vi "GUI Final add.vi"() -> ()   [LabVIEW 2014]
uses:
  <vilib>/Instr/_visa.llb/VISA Configure Serial Port (Instr).vi
panel:
  out "pass ACK":bool
  out "Threshold sent":bool
  out "no of trials read":bool
  out "PC on Ack":bool
  out "Reset#":i32
  in  "Reset":bool
  out "return count read":u32
  in  "VISA resource name":refnum<visa-resource-name>
  out "Iteration":i32
  in  "Tab Control":enum32{"Page 1", "Page 2", "Page 3"}(tab)
  in  "Password":string
  in  "Threshold":string
  out "read buffer":string
  out "password is wrong":bool
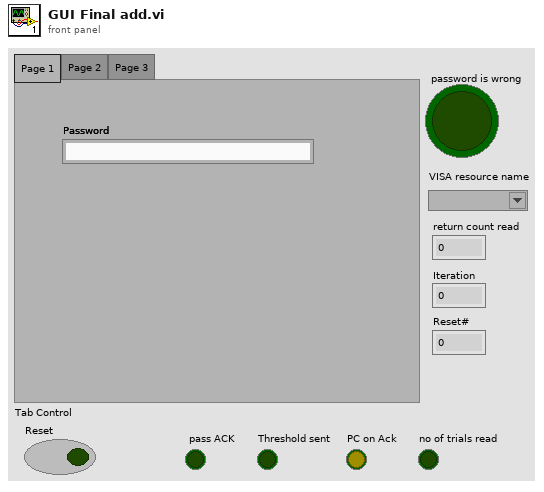
[diagram p1: front panel]
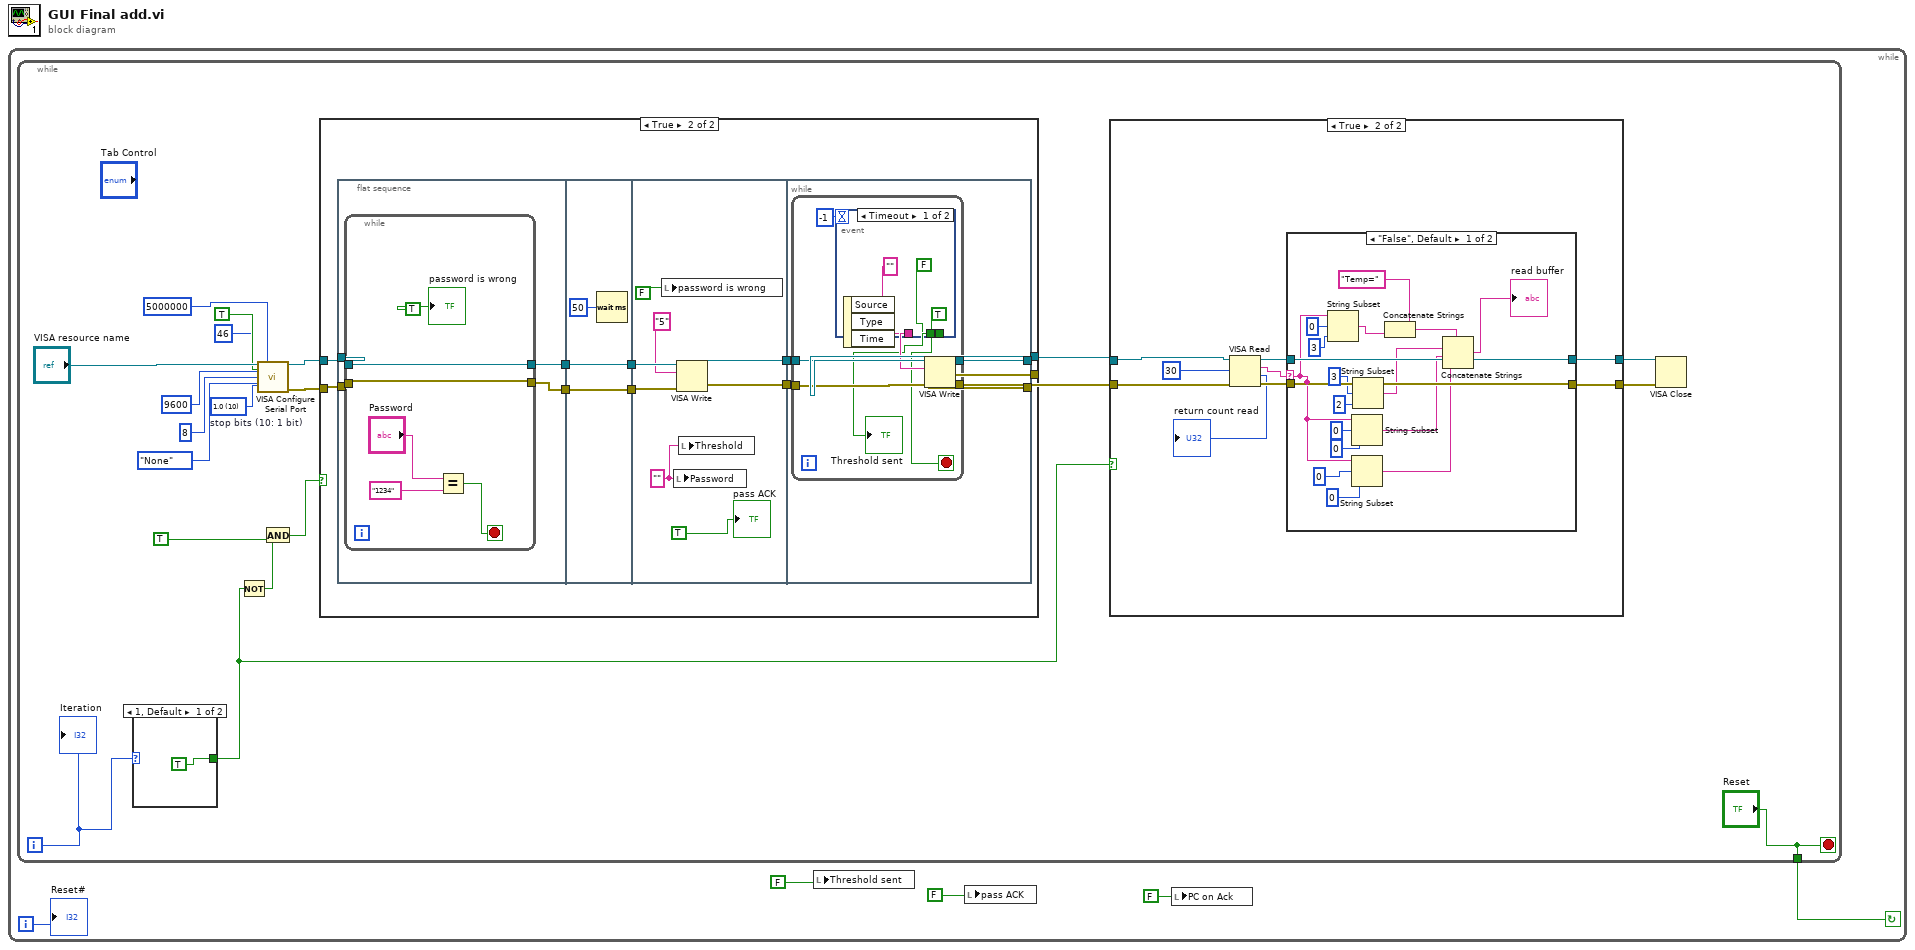
[diagram p0: block diagram]
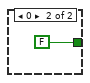
[diagram p2: hidden frame]
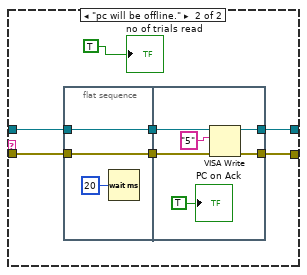
[diagram p4: hidden frame]
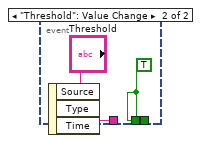
[diagram p6: hidden frame]
diagram:
  n1 = while {
    i -> [w5]
    stop <- w4 continue-if-true
    n2 = while {
      tunnel: ["Reset"] -> w4
      i -> [w9]
      stop <- "Reset" stop-if-true
      w22 = u16 10 items=["1.0"=10, "1.5"=15, "2.0"=20]  # stop bits (10: 1 bit)
      n3 = case shown="1, Default" w9 {
        tunnel: [TRUE FALSE] -> w8
        frame 1, Default {
        }
        frame 0 {
        }
      }
      n4 = Not(x=w8) -> (.not. x?=w17:bool)
      n5 = call-poly "VISA Configure Serial Port"("VISA resource name"="VISA resource name", "timeout (10sec)"=u32 5000000, "termination char\n(0xA = '\\n' = LF)"=u8 46 ("termination char\n(0xA = '\\n' = LF)"), "Enable Termination\nChar (T)"=TRUE ("Enable Termination\nChar (T)"), "baud rate (9600)"=u32 9600, "data bits (8)"=u16 8, "parity (0:none)"=enum16{"None", "Odd", "Even", "Mark", "Space"}."None", "stop bits (10: 1 bit)"=w22) -> ("VISA resource name out"=w16:refnum<visa-resource-name>, "error out"=w15:errorcluster)  [unwired: 6 in]
      n6 = And(x=w17, y=TRUE) -> (x .and. y?=w14:bool)
      n7 = case shown="True" w14 {
        tunnel: w15 -> [w74 w84]
        tunnel: [w73 w82] -> w13
        tunnel: [w74 w81] -> w11
        tunnel: w16 -> [w73 w83]
        frame False {
        }
        frame True {
          n8 = flat-sequence {
            tunnel: w84 -> [w88]
            tunnel: w83 -> [w87]
            tunnel: [w86] -> w78
            tunnel: [w85] -> w76
            tunnel: w78 -> [w97]
            tunnel: [w97] -> w77
            tunnel: w76 -> [w96]
            tunnel: [w96] -> w75
            tunnel: w77 -> [w105]
            tunnel: w75 -> [w104]
            tunnel: [w103] -> w80
            tunnel: [w102] -> w79
            tunnel: [w108] -> w82
            tunnel: [w107] -> w81
            tunnel: w80 -> [w109]
            tunnel: w79 -> [w106]
            frame #0 {
              n9 = while {
                tunnel: w88 -> [w93]
                tunnel: w87 -> [w92]
                tunnel: [w93] -> w86
                tunnel: [w92] -> w85
                stop <- w94 stop-if-true
                n10 = Equal?(x="Password", y="1234") -> (x = y?=w94:bool)
                "password is wrong" <- TRUE
              }
            }
            frame #1 {
              n11 = Wait (ms)(milliseconds to wait=u32 50) -> ()  [unwired: 1 out]
            }
            frame #2 {
              w99 = "" ("Password")
              n12 = local write "password is wrong"(FALSE) -> ()
              n13 = local write "Password"(w99) -> ()
              n14 = VISA Write(VISA resource name=w104, write buffer="5", error in (no error)=w105) -> (VISA resource name out=w103:refnum<visa-resource-name>, error out=w102:errorcluster)  [unwired: 1 out]
              n15 = local write "Threshold"(w99) -> ()
              "pass ACK" <- TRUE ("Pass Ack")
            }
            frame #3 {
              n16 = while {
                tunnel: w109 -> [w117]
                tunnel: [w116] -> w108
                tunnel: [w115] -> w107
                tunnel: w106 -> [w114]
                stop <- w111 stop-if-true
                n17 = event shown="[0] Timeout" {
                  selector: _ -> [_ _]
                  dyn-events: _ -> [_ _]
                  timeout: -1 -> [_ _]
                  tunnel: [TRUE w121] -> w111
                  tunnel: ["" "Threshold"] -> w113
                  tunnel: [FALSE w121] -> w110
                  event Timeout {
                    n18 = event-data() -> ()  [unwired: 1 in, 3 out]
                  }
                  event "Threshold": Value Change {
                    w121 = TRUE
                    n19 = event-data() -> ()  [unwired: 1 in, 3 out]
                  }
                }
                "Threshold sent" <- w110
                n20 = VISA Write(VISA resource name=w117, write buffer=w113, error in (no error)=w114) -> (VISA resource name out=w116:refnum<visa-resource-name>, error out=w115:errorcluster)  [unwired: 1 out]
              }
            }
          }
        }
      }
      n21 = case shown="True" w8 {
        tunnel: [w29 w37] -> w12
        tunnel: [w28 w38] -> w10
        tunnel: w13 -> [w29 w32]
        tunnel: w11 -> [w28 w31]
        frame False {
        }
        frame True {
          n22 = VISA Read(VISA resource name=w32, byte count=u32 30, error in (no error)=w31) -> (VISA resource name out=w35:refnum<visa-resource-name>, read buffer=w33:string, return count=→"return count read":u32, error out=w36:errorcluster)
          n23 = case shown="\"False\", Default" w33 {
            selector: w33 -> [w43 _]
            tunnel: [w55 w60] -> w38
            tunnel: [w56 w61] -> w37
            tunnel: w36 -> [w55 w62]
            tunnel: w35 -> [w56 w63]
            frame "False", Default {
              n24 = String Subset(string=w43, offset (0)=0, length (rest)=3 ("length (rest)")) -> (substring=w52:string)
              n25 = String Subset(string=w43, offset (0)=0, length (rest)=0 ("length (rest)")) -> (substring=w47:string)
              n26 = String Subset(string=w43, offset (0)=0, length (rest)=0 ("length (rest)")) -> (substring=w46:string)
              n27 = String Subset(string=w43, offset (0)=3, length (rest)=2 ("length (rest)")) -> (substring=w49:string)
              n28 = Concatenate Strings("Temp=" ("string"), w52) -> (w50:string)
              n29 = Concatenate Strings(w50, w49, w47, w46) -> (→"read buffer":string)
            }
            frame "pc will be offline." {
              n30 = flat-sequence {
                tunnel: w62 -> [w65]
                tunnel: w63 -> [w66]
                tunnel: [w66] -> w59
                tunnel: [w65] -> w58
                tunnel: [w70] -> w61
                tunnel: [w69] -> w60
                tunnel: w59 -> [w72]
                tunnel: w58 -> [w71]
                frame #0 {
                  n31 = Wait (ms)(milliseconds to wait=u32 20) -> ()  [unwired: 1 out]
                }
                frame #1 {
                  n32 = VISA Write(VISA resource name=w72, write buffer="5", error in (no error)=w71) -> (VISA resource name out=w70:refnum<visa-resource-name>, error out=w69:errorcluster)  [unwired: 1 out]
                  "PC on Ack" <- TRUE ("PC on Ack")
                }
              }
              "no of trials read" <- TRUE ("PC on Ack")
            }
          }
        }
      }
      n33 = VISA Close(VISA resource name=w12, error in (no error)=w10) -> ()  [unwired: 1 out]
      "Iteration" <- w9
    }
    n34 = local write "Threshold sent"(FALSE) -> ()
    n35 = local write "pass ACK"(FALSE ("Pass Ack")) -> ()
    n36 = local write "PC on Ack"(FALSE) -> ()
    "Reset#" <- w5
  }
